vi "StellarNet Get Spectrometer Coefficients from XML, ext precision.vi"(8 "error in (no error)":errorcluster, 11 "XML File Path":path) -> (0 "error out":errorcluster, 2 "file or folder exists?":bool, 3 "Multi Channel Coeffs & WLs":T1(array[cluster]))   [LabVIEW 2023]
uses:
  <vilib>/Utility/xml.llb/Read From XML File(string).vi
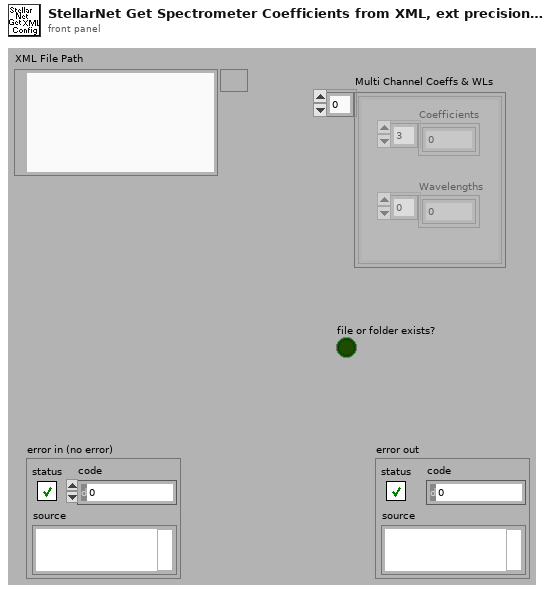
[diagram p1: front panel]
types:
  T1 = cluster{"Coefficients":ext[], "Wavelengths":dbl[]}[]
  T2 = cluster{"Coefficients":dbl[], "Wavelengths":dbl[]}[]
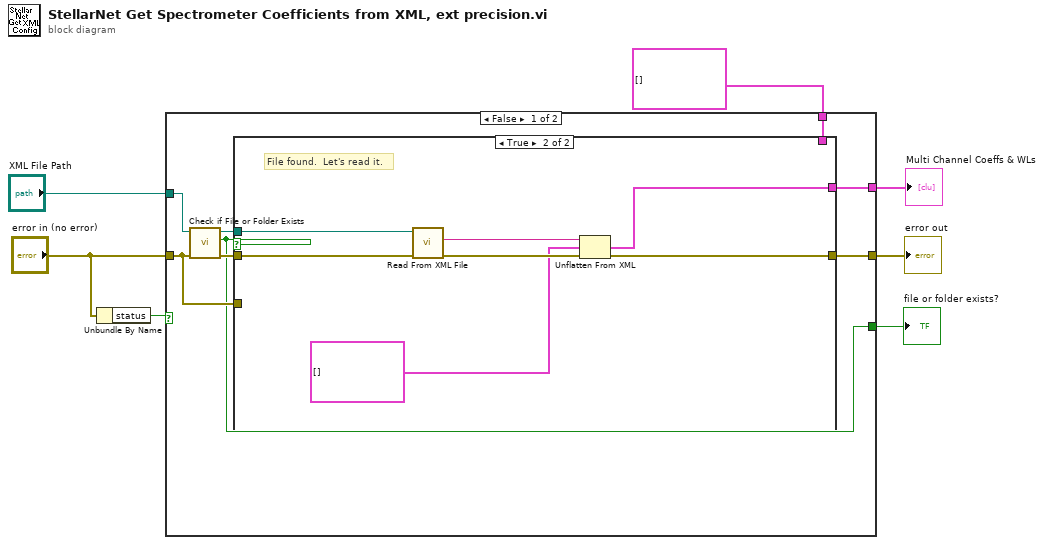
[diagram p0: block diagram]
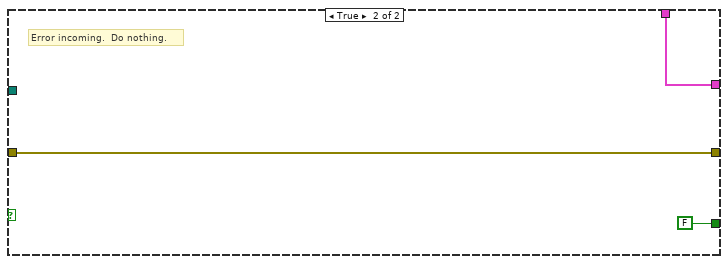
[diagram p3: hidden frame]
diagram:
  n1 = Unbundle By Name("error in (no error)") -> ("status"=w5:bool)
  n2 = case shown="False" w5 {
    tunnel: "XML File Path" -> [w15 _]
    tunnel: "error in (no error)" -> [w11 w27]
    tunnel: [w12 w27] -> w6
    tunnel: [w10 w25] -> w2
    tunnel: T2 [] ("Multi Channel Coeffs & WLs") -> [w9 w25]
    tunnel: [w8 FALSE ("file or folder exists?")] -> w3
    frame False {
      n3 = call <vilib>:"Check if File or Folder Exists.vi"("error in (no error)"=w11, "path"=w15) -> ("error out"=w14:errorcluster, "file or folder exists?"=w8:bool, "dup path"=w13:path)  [unwired: 7 in]
      n4 = case shown="True" w8 {
        tunnel: w14 -> [_ w22]
        tunnel: [w17 w21] -> w12
        tunnel: w13 -> [_ w20]
        tunnel: w11 -> [w17 _]
        tunnel: [w16 w19] -> w10
        tunnel: w9 -> [w16 _]
        frame False {
          # "File not found.  We'll create one later, so just pass the incoming error cluster through."
        }
        frame True {
          # "File found.  Let's read it."
          n5 = call-poly <vilib>:"Read From XML File.vi"("error in (no error)"=w22, "XML File Path"=w20) -> ("error out"=w23:errorcluster, "XML Elements"=w24:string)  [unwired: 7 in, 1 out]
          n6 = Unflatten From XML(xml string=w24, type=T2 [] ("Multi Channel Coeffs & WLs"), error in (no error)=w23) -> (value=w19:T2, error out=w21:errorcluster)
        }
      }
    }
    frame True {
      # "Error incoming.  Do nothing."
    }
  }
  "error out" <- w6
  "Multi Channel Coeffs & WLs" <- w2
  "file or folder exists?" <- w3
